vi "GetThermAlarmAnalogInputChannelAvailability.vi"(8 "error in":errorcluster, 10 "ThermAlarm number":T1=1 items=["ThermAlarm 1"=1, "ThermAlarm 2"=2, "ThermAlarm 3"=3, "ThermAlarm 4"=4], 11 "VISA resource name":refnum<visa-resource-name>) -> (0 "error out":errorcluster, 2 "analog input channel available?":i32, 3 "VISA resource name out":refnum<visa-resource-name>)   [LabVIEW 2023, in "Thermotron 8800.lvlib"]
doc: "ISAA\nCommand name: Send Therm-Alarm analog input channel availability\nCommand type: Variable\nDescription: The query command asks the 8800 if the analog input channel for Therm-Alarm “n” is available. The 8800 returns a 0 (not available) or a 1 (available).\nSyntax: ISAAn\nWhere n is a Therm-Alarm number (1 through 4).\nData type: Integer\nQuery example: ISAA1?\n8800 response: 1 (The analog input channel for Therm-Alarm 1 is available.)"
uses:
  Thermotron 8800.lvlib
  Private/ThermAlarmNumber.ctl
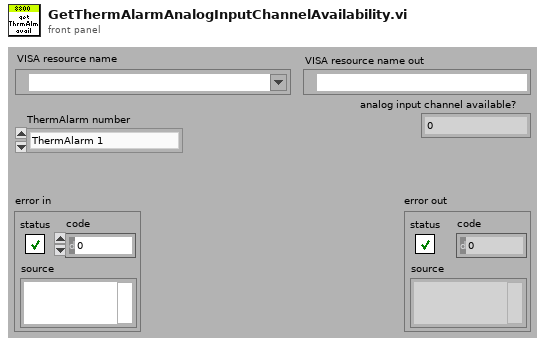
[diagram p1: front panel]
types:
  T1 = typedef "Thermotron 8800.lvlib/ThermAlarmNumber.ctl" = u16
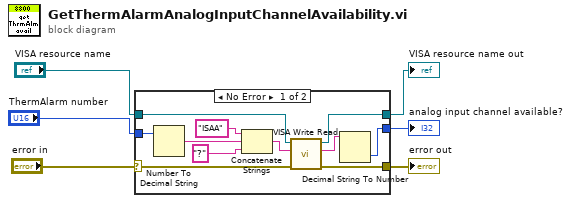
[diagram p0: block diagram]
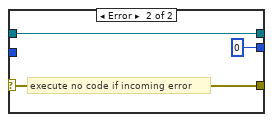
[diagram p2: hidden frame]
diagram:
  n1 = case shown="No Error" "error in" {
    selector: "error in" -> [w16 w20]
    tunnel: [w14 w20] -> w4
    tunnel: [w15 w19] -> w3
    tunnel: "VISA resource name" -> [w12 w19]
    tunnel: "ThermAlarm number" -> [w10 _]
    tunnel: [w7 0] -> w1
    frame No Error {
      n2 = Number To Decimal String(number=w10) -> (decimal integer string=w9:string)  [unwired: 1 in]
      n3 = Concatenate Strings("ISAA" ("8800 Command"), w9, "?" ("8800 Command")) -> (w17:string)
      n4 = call "VISA Write Read.vi"("error in (no error)"=w16, "8800 Command"=w17, "VISA Refnum in"=w12) -> ("error out"=w14:errorcluster, "read buffer"=w11:string, "VISA Refnum out"=w15:refnum<visa-resource-name>)  [unwired: 6 in]
      n5 = Decimal String To Number(string=w11) -> (number=w7:i32)  [unwired: 2 in, 1 out]
    }
    frame Error {
      # "execute no code if incoming error"
    }
  }
  "VISA resource name out" <- w3
  "error out" <- w4
  "analog input channel available?" <- w1
